vi "Do.vi"(7 "Mediated Asynchronous Actor":refnum<class "Mediated Asynchronous Actor.lvclass">, 8 "error in (no error)":errorcluster, 11 "Last Ack in":refnum<class "Last Ack.lvclass">) -> (0 "error out":errorcluster, 3 "Last Ack out":refnum<class "Last Ack.lvclass">, 5 "Mediated Asynchronous Actor out":refnum<class "Mediated Asynchronous Actor.lvclass">)   [LabVIEW 2016, in "Stream Mediator.lvlib" / "Last Ack.lvclass"]
doc: "--\nCopyright © 2017 Composed SystemsI All rights reserved.\n\nAuthor: Jon McBee <jon.mcbee@composed.io>\n\nThis library is provided \"AS IS\" ,WITHOUT WARRANTIES OR\nCONDITIONS OF ANY KIND, either express or implied.\n\nComposed Systems -- composed.io\n\nStream 0.0.1.1\nJon McBee - Composed Systems\nCopyright (c) 2017, Composed Systems"
uses:
  <userlib>/Composed Systems/Stream/Mediator/Classes/Message Command Last Ack/Last Ack.lvclass
  <userlib>/Composed Systems/Stream/Mediator/Classes/Mediated Asynchronous Actor/Mediated Asynchronous Actor.lvclass
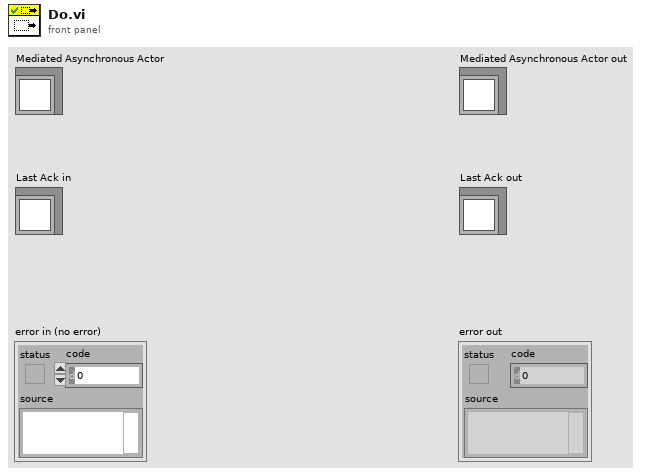
[diagram p1: front panel]
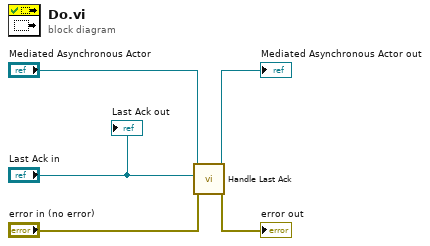
[diagram p0: block diagram]
diagram:
  n1 = call <userlib>:"Handle Last Ack.vi"("error in (no error)"="error in (no error)", "Last Ack"="Last Ack in", "Mediated Asynchronous Actor in"="Mediated Asynchronous Actor") -> ("error out"=→"error out":errorcluster, "Mediated Asynchronous Actor out"=→"Mediated Asynchronous Actor out":refnum<class "Mediated Asynchronous Actor.lvclass">)  [unwired: 7 in]
  "Last Ack out" <- "Last Ack in"
